vi "ActionVIOnDownload_LaunchDaemon.vi"(5 "System Definition Dir":path, 6 "IP address":string, 7 "Details Ref":refnum<vi>, 8 "error in (no error)":errorcluster, 10 "WebDAV session in":T1, 11 "Device Item Ref in":T2 format="%.0x") -> (0 "error out":errorcluster, 2 "WebDAV session out":T1, 3 "Device Item Ref out":T2 format="%.0x")   [LabVIEW 2015, in "Host Heartbeat System Explorer.lvlib"]
uses:
  Host Heartbeat System Explorer.lvlib
  <vilib>/NI Veristand/Custom Device API/Custom Device Item Ref.ctl
  <vilib>/WebDAVClient/Advanced/SessionHandle.ctl
  Shared/Constants.vi
  <vilib>/NI Veristand/Custom Device API/Get Item Property (U16).vi
  <vilib>/NI Veristand/Custom Device API/Custom Device API.lvlib
  Shared/Host Heartbeat Shared.lvlib
  <vilib>/WebDAVClient/NI_WebDAV.lvlib
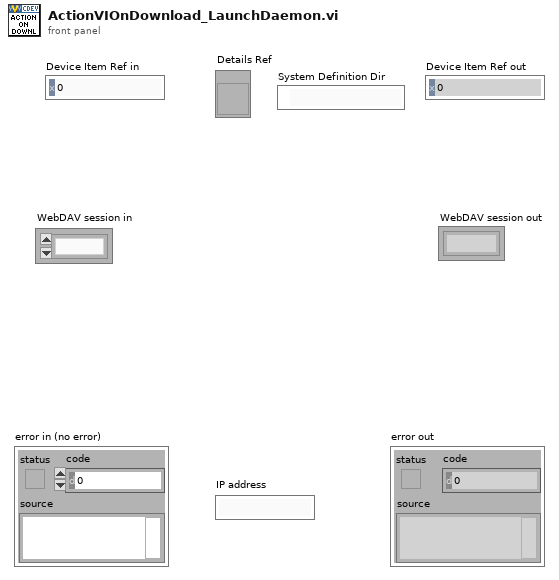
[diagram p1: front panel]
types:
  T1 = typedef "NI_WebDAV.lvlib/SessionHandle.ctl" = refnum<k1>
  T2 = typedef "Custom Device API.lvlib/Custom Device Item Ref.ctl" = u64
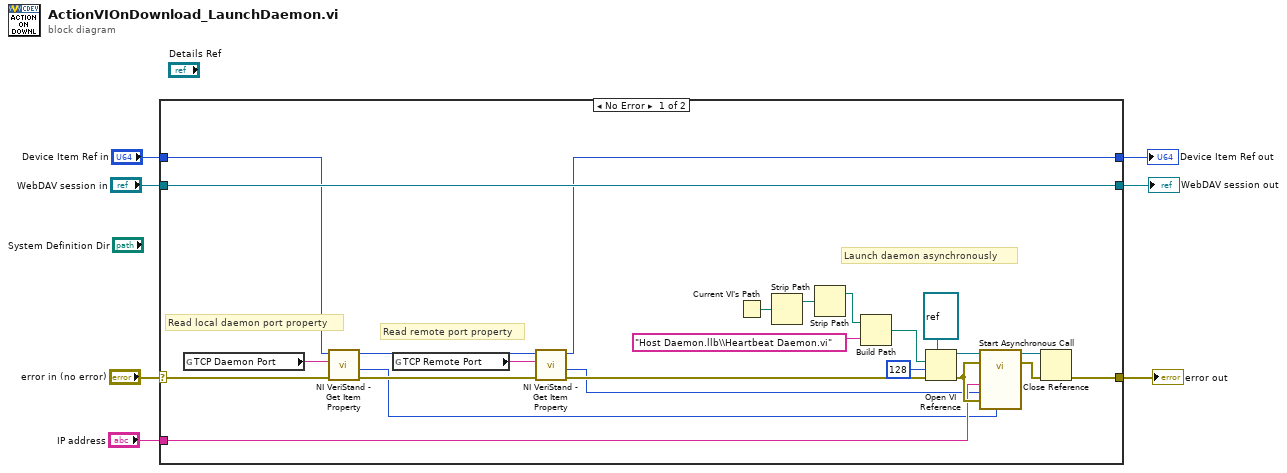
[diagram p0: block diagram]
diagram:
  n1 = case shown="No Error" "error in (no error)" {
    selector: "error in (no error)" -> [w17 w34]
    tunnel: [w24 w34] -> w6
    tunnel: "WebDAV session in" -> [w31 w33]
    tunnel: [w31 w33] -> w2
    tunnel: "Device Item Ref in" -> [w18 w32]
    tunnel: [w10 w32] -> w4
    tunnel: "IP address" -> [w19 _]
    frame No Error {
      # "Read local daemon port property"
      # "Launch daemon asynchronously"
      # "Read remote port property"
      n2 = global read "Constants.vi" "TCP Daemon Port"() -> (w16:string)
      n3 = call-poly <vilib>:"NI VeriStand - Get Item Property.vi"("error in (no error)"=w17, "Property Name"=w16, "Item Ref in"=w18) -> ("error out"=w13:errorcluster, "Value"=w8:u16, "Item Ref out"=w11:T2)  [unwired: 5 in, 1 out]
      n4 = global read "Constants.vi" "TCP Remote Port"() -> (w14:string)
      n5 = call-poly <vilib>:"NI VeriStand - Get Item Property.vi"("error in (no error)"=w13, "Property Name"=w14, "Item Ref in"=w11) -> ("error out"=w12:errorcluster, "Value"=w9:u16, "Item Ref out"=w10:T2)  [unwired: 5 in, 1 out]
      n6 = Current VI's Path() -> (path=w22:path)
      n7 = Strip Path(path=w22) -> (stripped path=w21:path)  [unwired: 1 out]
      n8 = Strip Path(path=w21) -> (stripped path=w20:path)  [unwired: 1 out]
      n9 = Build Path(base path=w20, name or relative path="Host Daemon.llb\\Heartbeat Daemon.vi") -> (appended path=w23:path)
      n10 = Open VI Reference(type specifier VI Refnum (for type only)=refnum<vi> refnum, vi path=w23, options=128, error in (no error)=w12) -> (vi reference=w29:refnum<vi>, error out=w27:errorcluster)  [unwired: 2 in]
      n11 = call-by-ref "Start Asynchronous Call"(reference=w29, error in=w27, "Local Daemon Port"=w8, "Error In"=w27, "Remote Port"=w9, "Target IP"=w19) -> (reference out=w25:refnum<vi>, error out=w26:errorcluster)  [unwired: 8 in]
      n12 = Close Reference(reference=w25, error in (no error)=w26) -> (error out=w24:errorcluster)
    }
    frame Error {
    }
  }
  "error out" <- w6
  "Device Item Ref out" <- w4
  "WebDAV session out" <- w2
